vi "LabMat3MAT.vi"(2 "replace source":T1, 4 "error in (no error)":errorcluster, 5 "b":cluster{i32, i32}(slide)={-21, 6} scale=-50.0..50.0, 6 "a":cluster{i32, i32}(slide)={-21, -7} scale=-50.0..50.0, 7 "L":cluster{i32, i32}(slide)={81, 99} scale=0.0..100.0, 11 "Image":T1) -> (0 "error out":errorcluster, 3 "Image  output":T1(plugin-control), 8 "Histogram 3":dynamicdata(graph) caption="B直方图", 9 "Histogram 2":dynamicdata(graph) caption="A直方图", 10 "Histogram":dynamicdata(graph) caption="L直方图")   [LabVIEW 2018]
uses:
  <vilib>/vision/Image Controls.llb/IMAQ Image.ctl
  <vilib>/vision/NI_Vision_Development_Module.lvlib
panel:
  out "B":u8[][](array[numeric])
  out "列":i32
  out "行":i32
  out "G":u8[][](array[numeric])
  out "R":u8[][](array[numeric])
  # "sourece"
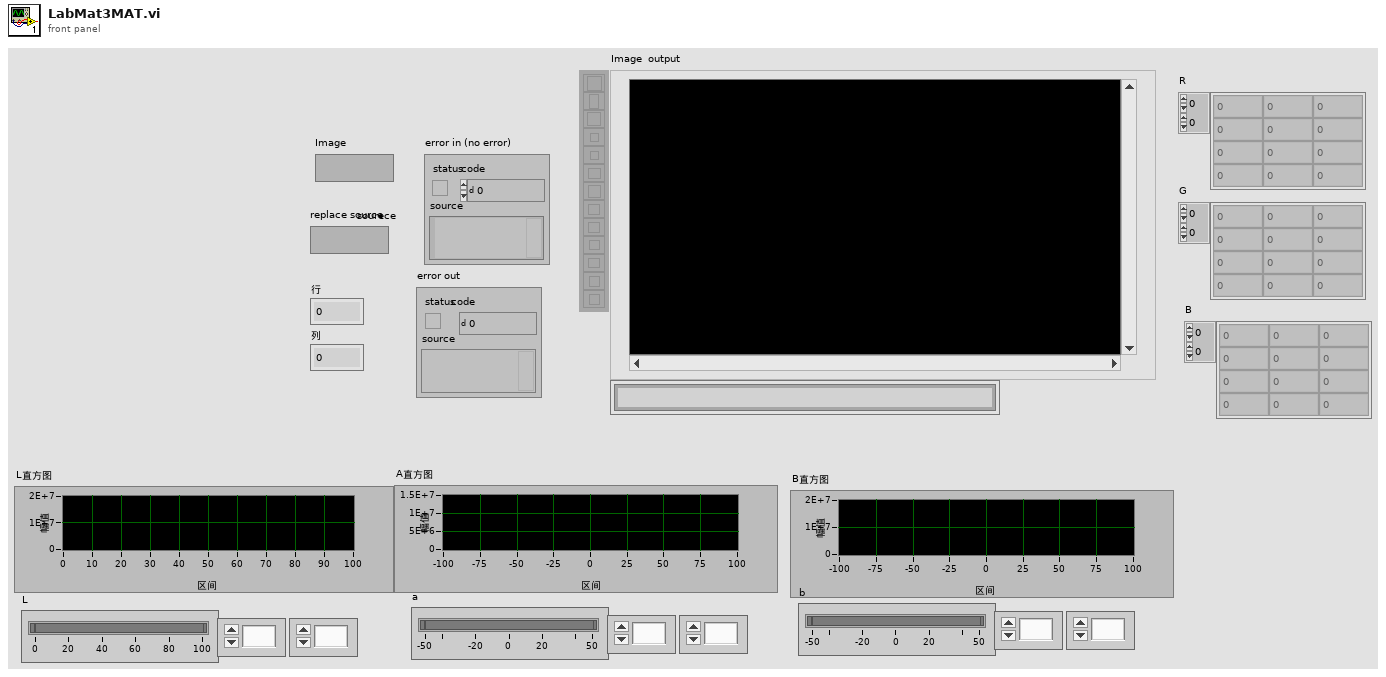
[diagram p1: front panel]
types:
  T1 = typedef "IMAQ Image.ctl" = refnum<image>
  T2 = typedef "Image Type" = u32
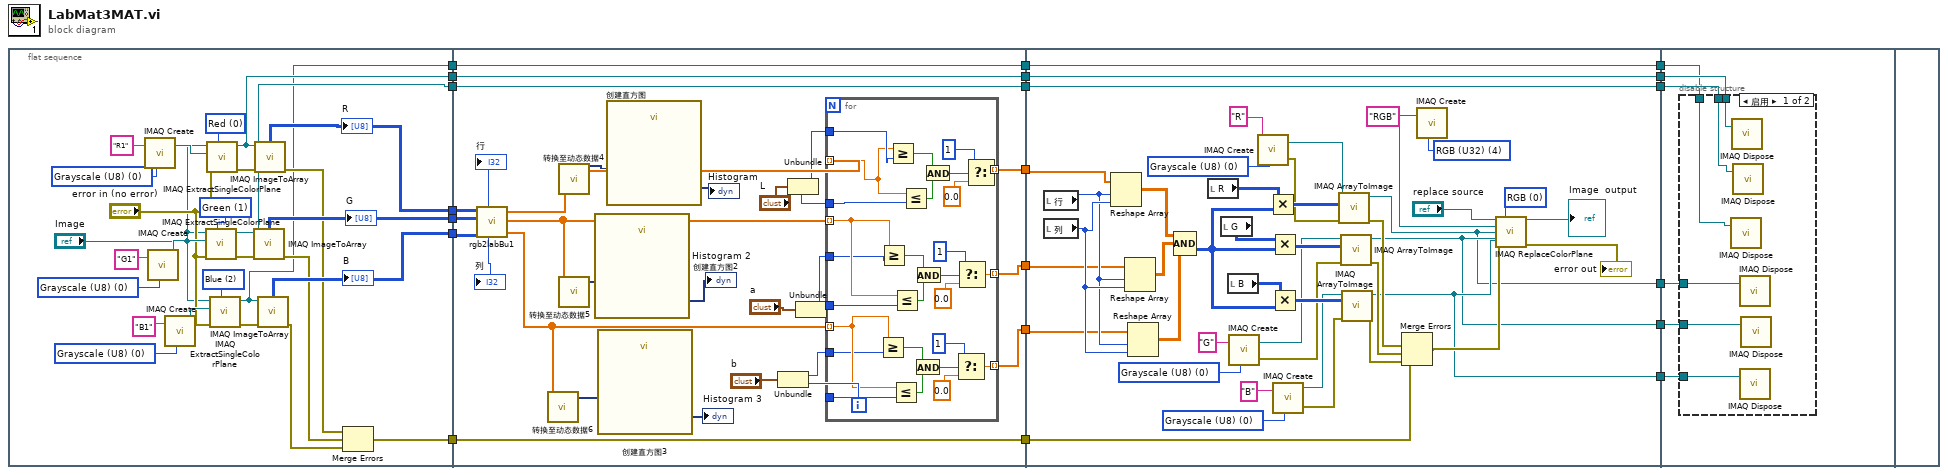
[diagram p0: block diagram]
diagram:
  n1 = flat-sequence {
    tunnel: [w47] -> w20
    tunnel: [w46] -> w19
    tunnel: [w45] -> w18
    tunnel: [w41] -> w17
    tunnel: [w40] -> w10
    tunnel: [w39] -> w7
    tunnel: [w38] -> w4
    tunnel: w20 -> [w57]
    tunnel: w19 -> [w56]
    tunnel: w18 -> [w55]
    tunnel: w17 -> [w54]
    tunnel: [w54] -> w16
    tunnel: [w53] -> w15
    tunnel: [w52] -> w14
    tunnel: [w51] -> w13
    tunnel: [w50] -> w11
    tunnel: w10 -> [w50]
    tunnel: [w49] -> w8
    tunnel: w7 -> [w49]
    tunnel: [w48] -> w5
    tunnel: w4 -> [w48]
    tunnel: w16 -> [w115]
    tunnel: w15 -> [w114]
    tunnel: w14 -> [w113]
    tunnel: w13 -> [w112]
    tunnel: [w111] -> w12
    tunnel: w11 -> [w111]
    tunnel: [w110] -> w9
    tunnel: w8 -> [w110]
    tunnel: [w109] -> w6
    tunnel: w5 -> [w109]
    tunnel: [w107] -> w3
    tunnel: [w106] -> w2
    tunnel: [w105] -> w1
    tunnel: w12 -> [w155]
    tunnel: w9 -> [w154]
    tunnel: w6 -> [w153]
    tunnel: w3 -> [w152]
    tunnel: w2 -> [w151]
    tunnel: w1 -> [w150]
    frame #0 {
      w26 = 2 items=["Red", "Green", "Blue", "Hue", "Saturation", "Luminance", "Value", "Intensity"] ("Color Plane")
      w27 = 1 items=["Red", "Green", "Blue", "Hue", "Saturation", "Luminance", "Value", "Intensity"] ("Color Plane")
      w28 = 0 items=["Red", "Green", "Blue", "Hue", "Saturation", "Luminance", "Value", "Intensity"] ("Color Plane")
      w32 = T2 0 items=["Grayscale (U8)", "Grayscale (I16)", "Grayscale (SGL)", "Complex (CSG)", "RGB (U32)", "HSL (U32)", "RGB (U64)", "Grayscale (U16)"] ("Image Type")
      w34 = T2 0 items=["Grayscale (U8)", "Grayscale (I16)", "Grayscale (SGL)", "Complex (CSG)", "RGB (U32)", "HSL (U32)", "RGB (U64)", "Grayscale (U16)"] ("Image Type")
      w36 = T2 0 items=["Grayscale (U8)", "Grayscale (I16)", "Grayscale (SGL)", "Complex (CSG)", "RGB (U32)", "HSL (U32)", "RGB (U64)", "Grayscale (U16)"] ("Image Type")
      n2 = call "IMAQ Create"("Image Name"="R1", "Image Type"=w36) -> ("New Image"=w31:T1)  [unwired: 2 in, 2 out]
      n3 = call "IMAQ Create"("Image Name"="G1", "Image Type"=w34) -> ("New Image"=w30:T1)  [unwired: 2 in, 2 out]
      n4 = call "IMAQ Create"("Image Name"="B1", "Image Type"=w32) -> ("New Image"=w29:T1)  [unwired: 2 in, 2 out]
      n5 = call "IMAQ ExtractSingleColorPlane"("Color Plane"=w27, "error in (no error)"="error in (no error)", "Image Dst"=w30, "Image Src"="Image") -> ("error out"=w24:errorcluster, "Image Dst Out"=w39:T1)  [unwired: 6 in]
      n6 = call "IMAQ ExtractSingleColorPlane"("Color Plane"=w28, "error in (no error)"="error in (no error)", "Image Dst"=w31, "Image Src"="Image") -> ("error out"=w25:errorcluster, "Image Dst Out"=w40:T1)  [unwired: 6 in]
      n7 = call "IMAQ ExtractSingleColorPlane"("Color Plane"=w26, "error in (no error)"="error in (no error)", "Image Dst"=w29, "Image Src"="Image") -> ("error out"=w22:errorcluster, "Image Dst Out"=w38:T1)  [unwired: 6 in]
      n8 = call "IMAQ ImageToArray"("error in (no error)"=w24, "Image"=w39) -> ("error out"=w43:errorcluster, "Image Pixels (U8)"=w46:u8[][])  [unwired: 2 in, 3 out]
      "G" <- w46
      n9 = call "IMAQ ImageToArray"("error in (no error)"=w25, "Image"=w40) -> ("error out"=w44:errorcluster, "Image Pixels (U8)"=w47:u8[][])  [unwired: 2 in, 3 out]
      "R" <- w47
      n10 = call "IMAQ ImageToArray"("error in (no error)"=w22, "Image"=w38) -> ("error out"=w42:errorcluster, "Image Pixels (U8)"=w45:u8[][])  [unwired: 2 in, 3 out]
      "B" <- w45
      n11 = Merge Errors(w44, w43, w42) -> (w41:errorcluster)
    }
    frame #1 {
      n12 = call "rgb2labBu1.vi"("R"=w57, "G"=w56, "B"=w55) -> ("hang"=→"行":i32, "lie"=→"列":i32, "LZ"=w73:dbl[], "aZ"=w74:dbl[], "bZ"=w75:dbl[])  [unwired: 1 in]
      n13 = call "转换至动态数据6"("Array"=w75) -> ("Dynamic Data Type"=w60:dynamicdata)  [unwired: 3 in]
      n14 = call "转换至动态数据4"("Array"=w73) -> ("Dynamic Data Type"=w58:dynamicdata)  [unwired: 3 in]
      n15 = call "转换至动态数据5"("Array"=w74) -> ("Dynamic Data Type"=w59:dynamicdata)  [unwired: 3 in]
      n16 = call "创建直方图2"("Signal"=w59) -> ("Histogram"=→"Histogram 2":dynamicdata)  [unwired: 9 in, 1 out]
      n17 = call "创建直方图3"("Signal"=w60) -> ("Histogram"=→"Histogram 3":dynamicdata)  [unwired: 9 in, 1 out]
      n18 = call "创建直方图"("Signal"=w58) -> ("Histogram"=→"Histogram":dynamicdata)  [unwired: 9 in, 1 out]
      n19 = Unbundle("b") -> (w71:i32, w72:i32)
      n20 = Unbundle("L") -> (w67:i32, w68:i32)
      n21 = Unbundle("a") -> (w69:i32, w70:i32)
      n22 = for {
        tunnel: w73 -> [w97] mode=indexing
        tunnel: w67 -> [w99]
        tunnel: w68 -> [w100]
        tunnel: [w101] -> w53 mode=indexing
        tunnel: w74 -> [w85] mode=indexing
        tunnel: w75 -> [w84] mode=indexing
        tunnel: w69 -> [w83]
        tunnel: w70 -> [w82]
        tunnel: w71 -> [w81]
        tunnel: w72 -> [w80]
        tunnel: [w79] -> w52 mode=indexing
        tunnel: [w78] -> w51 mode=indexing
        n23 = Greater Or Equal?(x=w84, y=w81) -> (x >= y?=w90:bool)
        n24 = Greater Or Equal?(x=w85, y=w83) -> (x >= y?=w95:bool)
        n25 = Greater Or Equal?(x=w97, y=w99) -> (x >= y?=w104:bool)
        n26 = Less Or Equal?(x=w84, y=w80) -> (x <= y?=w89:bool)
        n27 = Less Or Equal?(x=w85, y=w82) -> (x <= y?=w94:bool)
        n28 = Less Or Equal?(x=w97, y=w100) -> (x <= y?=w103:bool)
        n29 = And(x=w90, y=w89) -> (x .and. y?=w88:bool)
        n30 = And(x=w95, y=w94) -> (x .and. y?=w93:bool)
        n31 = And(x=w104, y=w103) -> (x .and. y?=w102:bool)
        n32 = Select(t=1, s=w88, f=0.0) -> (s? t:f=w78:dbl)
        n33 = Select(t=1, s=w93, f=0.0) -> (s? t:f=w79:dbl)
        n34 = Select(t=1, s=w102, f=0.0) -> (s? t:f=w101:dbl)
      }
    }
    frame #2 {
      w147 = u16 0 items=["RGB", "HSL", "HSV", "HSI"] ("Color Mode")
      w138 = T2 4 items=["Grayscale (U8)", "Grayscale (I16)", "Grayscale (SGL)", "Complex (CSG)", "RGB (U32)", "HSL (U32)", "RGB (U64)", "Grayscale (U16)"] ("Image Type")
      w123 = T2 0 items=["Grayscale (U8)", "Grayscale (I16)", "Grayscale (SGL)", "Complex (CSG)", "RGB (U32)", "HSL (U32)", "RGB (U64)", "Grayscale (U16)"] ("Image Type")
      w121 = T2 0 items=["Grayscale (U8)", "Grayscale (I16)", "Grayscale (SGL)", "Complex (CSG)", "RGB (U32)", "HSL (U32)", "RGB (U64)", "Grayscale (U16)"] ("Image Type")
      w117 = T2 0 items=["Grayscale (U8)", "Grayscale (I16)", "Grayscale (SGL)", "Complex (CSG)", "RGB (U32)", "HSL (U32)", "RGB (U64)", "Grayscale (U16)"] ("Image Type")
      n35 = local read "行"() -> (w139:i32)
      n36 = local read "列"() -> (w140:i32)
      n37 = Reshape Array(w114, w139, w140) -> (w141:dbl[][])
      n38 = Reshape Array(w113, w139, w140) -> (w142:dbl[][])
      n39 = Reshape Array(w112, w139, w140) -> (w143:dbl[][])
      n40 = Compound Arithmetic op=AND(w141, w142, w143) -> (w144:i32[][])
      n41 = local read "R"() -> (w128:u8[][])
      n42 = local read "G"() -> (w129:u8[][])
      n43 = local read "B"() -> (w146:u8[][])
      n44 = call "IMAQ Create"("Image Name"="G", "Image Type"=w121) -> ("New Image"=w124:T1, "error out"=w125:errorcluster)  [unwired: 2 in, 1 out]
      n45 = call "IMAQ Create"("Image Name"="R", "Image Type"=w117) -> ("New Image"=w118:T1, "error out"=w119:errorcluster)  [unwired: 2 in, 1 out]
      n46 = Multiply(x=w128, y=w144) -> (x*y=w130:i32[][])
      n47 = Multiply(x=w129, y=w144) -> (x*y=w131:i32[][])
      n48 = Multiply(x=w146, y=w144) -> (x*y=w132:i32[][])
      n49 = call "IMAQ Create"("Image Name"="B", "Image Type"=w123) -> ("New Image"=w126:T1, "error out"=w127:errorcluster)  [unwired: 2 in, 1 out]
      n50 = call "IMAQ ArrayToImage"("error in (no error)"=w119, "Image Pixels (U8)"=w130, "Image"=w118) -> ("error out"=w133:errorcluster, "Image Out"=w105:T1)  [unwired: 7 in]
      n51 = call "IMAQ ArrayToImage"("error in (no error)"=w125, "Image Pixels (U8)"=w131, "Image"=w124) -> ("error out"=w134:errorcluster, "Image Out"=w106:T1)  [unwired: 7 in]
      n52 = call "IMAQ ArrayToImage"("error in (no error)"=w127, "Image Pixels (U8)"=w132, "Image"=w126) -> ("error out"=w135:errorcluster, "Image Out"=w107:T1)  [unwired: 7 in]
      n53 = Merge Errors(w115, w133, w134, w135) -> (w136:errorcluster)
      n54 = call "IMAQ Create"("Image Name"="RGB", "Image Type"=w138) -> ("New Image"=w145:T1)  [unwired: 2 in, 2 out]
      n55 = call "IMAQ ReplaceColorPlane"("Image Src"="replace source", "Color Mode"=w147, "Image Dst"=w145, "Red or Hue Plane"=w105, "Green or Sat Plane"=w106, "error in (no error)"=w136, "Blue or Luma or Val or Inten Plane"=w107) -> ("Image Dst Out"=→"Image  output":T1, "error out"=→"error out":errorcluster)  [unwired: 7 in]
    }
    frame #3 {
      n56 = disable-structure shown="启用" {
        disable-tunnel: w155 -> [w161 _]
        disable-tunnel: w154 -> [w160 _]
        disable-tunnel: w153 -> [w159 _]
        disable-tunnel: w152 -> [w158 _]
        disable-tunnel: w151 -> [w157 _]
        disable-tunnel: w150 -> [w156 _]
        frame Enabled {
          n57 = call "IMAQ Dispose"("Image"=w159) -> ()  [unwired: 5 in, 1 out]
          n58 = call "IMAQ Dispose"("Image"=w161) -> ()  [unwired: 5 in, 1 out]
          n59 = call "IMAQ Dispose"("Image"=w160) -> ()  [unwired: 5 in, 1 out]
          n60 = call "IMAQ Dispose"("Image"=w156) -> ()  [unwired: 5 in, 1 out]
          n61 = call "IMAQ Dispose"("Image"=w158) -> ()  [unwired: 5 in, 1 out]
          n62 = call "IMAQ Dispose"("Image"=w157) -> ()  [unwired: 5 in, 1 out]
        }
        frame Disabled {
        }
      }
    }
    frame #4 {
    }
  }
